vi "sv_Configure MSG for Triggered Signals with Limits.vi"(8 "error in (no error)":errorcluster, 10 "number of response channels":i32=1, 11 "MSG reference in":refnum<vi>) -> (0 "error out":errorcluster, 3 "MSG reference out":refnum<vi>)   [LabVIEW 2017]
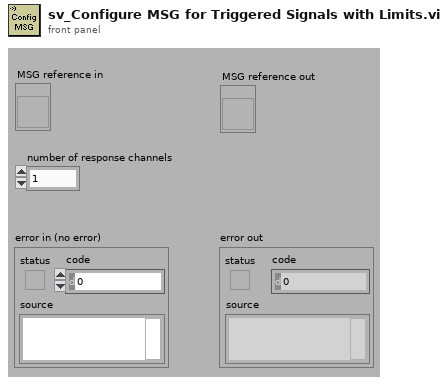
[diagram p1: front panel]
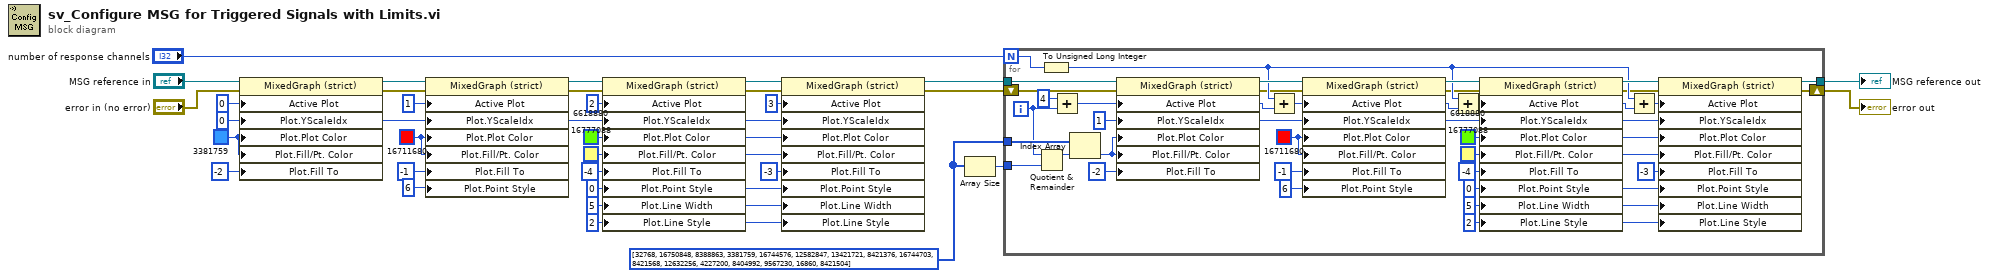
[diagram p0: block diagram]
diagram:
  w2 = u32[] [32768, 16750848, 8388863, 3381759, 16744576, 12582847, 13421721, 8421376, 16744703, 8421568, 12632256, 4227200, 8404992, 9567230, 16860, 8421504]
  w29 = u32 16777088 ("Plot.Plot Color")
  w27 = u8 2 ("Plot.Line Style")
  w26 = u8 5 ("Plot.Line Width")
  w25 = u8 0 ("Plot.Point Style")
  w28 = u32 6618880 ("Plot.Plot Color")
  w16 = u32 16711680 ("Plot.Plot Color")
  w24 = u32 0 ("Plot.Y Scale Index")
  w11 = u32 3381759 ("Plot.Plot Color")
  n1 = property class="MixedGraph (strict)"(reference="MSG reference in", error in="error in (no error)", "Active Plot"=u32 0, "Plot.YScaleIdx"=w24, "Plot.Plot Color"=w11, "Plot.Fill/Pt. Color"=w11, "Plot.Fill To"=i16 -2) -> (reference out=w17:refnum<vi>, error out=w9:errorcluster)
  n2 = property class="MixedGraph (strict)"(reference=w17, error in=w9, "Active Plot"=u32 1, "Plot.YScaleIdx"=w24, "Plot.Plot Color"=w16, "Plot.Fill/Pt. Color"=w16, "Plot.Fill To"=i16 -1, "Plot.Point Style"=u8 6) -> (reference out=w21:refnum<vi>, error out=w8:errorcluster)
  n3 = property class="MixedGraph (strict)"(reference=w21, error in=w8, "Active Plot"=u32 2, "Plot.YScaleIdx"=w24, "Plot.Plot Color"=w28, "Plot.Fill/Pt. Color"=w29, "Plot.Fill To"=i16 -4, "Plot.Point Style"=w25, "Plot.Line Width"=w26, "Plot.Line Style"=w27) -> (reference out=w30:refnum<vi>, error out=w7:errorcluster)
  n4 = property class="MixedGraph (strict)"(reference=w30, error in=w7, "Active Plot"=u32 3, "Plot.YScaleIdx"=w24, "Plot.Plot Color"=w28, "Plot.Fill/Pt. Color"=w29, "Plot.Fill To"=i16 -3, "Plot.Point Style"=w25, "Plot.Line Width"=w26, "Plot.Line Style"=w27) -> (reference out=w4:refnum<vi>, error out=w6:errorcluster)
  n5 = Array Size(array=w2) -> (size(s)=w1:i32)
  n6 = for {
    N: "number of response channels" -> [w48]
    tunnel: w2 -> [w50]
    shift-right: [w38] -> w5
    shift-left: w6 -> [w39]
    tunnel: w4 -> [w51]
    tunnel: [w37] -> w3
    tunnel: w1 -> [w35]
    i -> [w33]
    w65 = u32 16777088 ("Plot.Plot Color")
    w63 = u8 2 ("Plot.Line Style")
    w62 = u8 5 ("Plot.Line Width")
    w61 = u8 0 ("Plot.Point Style")
    w64 = u32 6618880 ("Plot.Plot Color")
    w54 = u32 16711680 ("Plot.Plot Color")
    w60 = u32 1 ("Plot.Y Scale Index")
    n7 = Quotient & Remainder(x=w33, y=w35) -> (x-y*floor(x/y)=w34:i32)  [unwired: 1 out]
    n8 = To Unsigned Long Integer(number=w48) -> (unsigned 32bit integer=w46:u32)
    n9 = Add(x=u32 4, y=w33) -> (x+y=w44:u32)
    n10 = Index Array(array=w50, index=w34) -> (element=w36:u32)
    n11 = property class="MixedGraph (strict)"(reference=w51, error in=w39, "Active Plot"=w44, "Plot.YScaleIdx"=w60, "Plot.Plot Color"=w36, "Plot.Fill/Pt. Color"=w36, "Plot.Fill To"=i16 -2) -> (reference out=w55:refnum<vi>, error out=w45:errorcluster)
    n12 = Add(x=w46, y=w44) -> (x+y=w43:u32)
    n13 = property class="MixedGraph (strict)"(reference=w55, error in=w45, "Active Plot"=w43, "Plot.YScaleIdx"=w60, "Plot.Plot Color"=w54, "Plot.Fill/Pt. Color"=w54, "Plot.Fill To"=i16 -1, "Plot.Point Style"=u8 6) -> (reference out=w58:refnum<vi>, error out=w40:errorcluster)
    n14 = Add(x=w46, y=w43) -> (x+y=w42:u32)
    n15 = property class="MixedGraph (strict)"(reference=w58, error in=w40, "Active Plot"=w42, "Plot.YScaleIdx"=w60, "Plot.Plot Color"=w64, "Plot.Fill/Pt. Color"=w65, "Plot.Fill To"=i16 -4, "Plot.Point Style"=w61, "Plot.Line Width"=w62, "Plot.Line Style"=w63) -> (reference out=w66:refnum<vi>, error out=w41:errorcluster)
    n16 = Add(x=w46, y=w42) -> (x+y=w47:u32)
    n17 = property class="MixedGraph (strict)"(reference=w66, error in=w41, "Active Plot"=w47, "Plot.YScaleIdx"=w60, "Plot.Plot Color"=w64, "Plot.Fill/Pt. Color"=w65, "Plot.Fill To"=i16 -3, "Plot.Point Style"=w61, "Plot.Line Width"=w62, "Plot.Line Style"=w63) -> (reference out=w37:refnum<vi>, error out=w38:errorcluster)
  }
  "MSG reference out" <- w3
  "error out" <- w5
